vi "Lab1_Exercise2.vi"() -> ()   [LabVIEW 2016]
panel:
  out "Boolean 6":bool
  in  "Boolean 5":bool
  in  "Boolean 4":bool
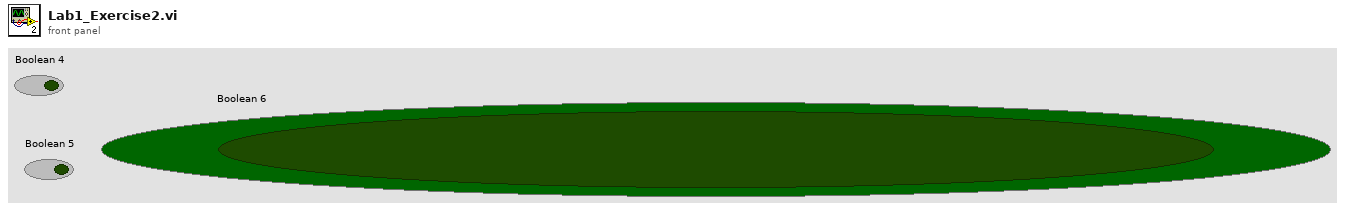
[diagram p1: front panel]
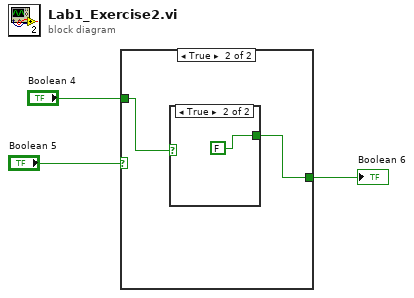
[diagram p0: block diagram]
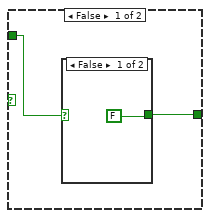
[diagram p2: hidden frame]
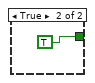
[diagram p3: hidden frame]
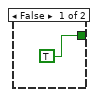
[diagram p4: hidden frame]
diagram:
  n1 = case shown="True" "Boolean 5" {
    tunnel: [w5 w9] -> w2
    tunnel: "Boolean 4" -> [w4 w8]
    frame False {
      n2 = case shown="False" w4 {
        tunnel: [FALSE TRUE] -> w5
        frame False {
        }
        frame True {
        }
      }
    }
    frame True {
      n3 = case shown="True" w8 {
        tunnel: [TRUE FALSE] -> w9
        frame False {
        }
        frame True {
        }
      }
    }
  }
  "Boolean 6" <- w2
